vi "DestroyRenderer.vi"(8 "No Error":errorcluster, 11 "Rrenderer [SDL_Renderer *]":i64 format="%.0x") -> (0 "error out":errorcluster)   [LabVIEW 2024, in "SDL3.lvlib" / "Render.lvlib"]
doc: "<B>Summary</B>\nDestroy the rendering context for a window and free all associated textures.\n\n<B>Remarks</B>\nThis should be called before destroying the associated window."
uses:
  Render.lvlib
  Lib/Win32/SDL3.dll
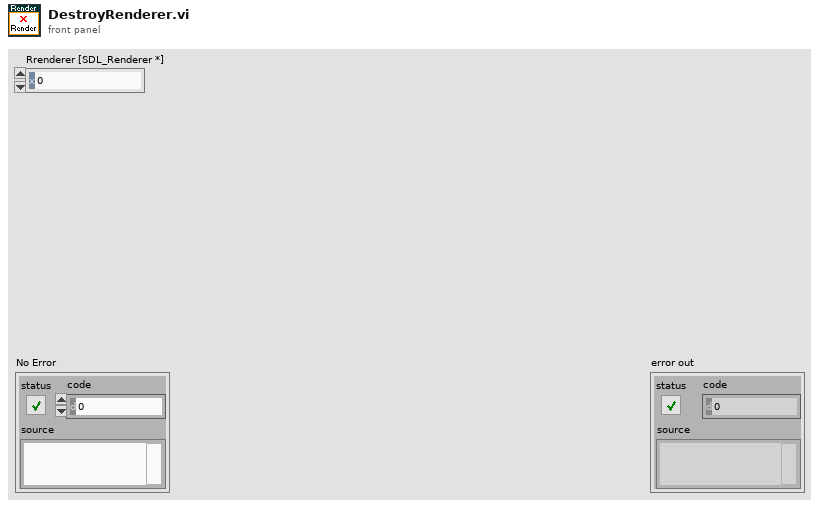
[diagram p1: front panel]
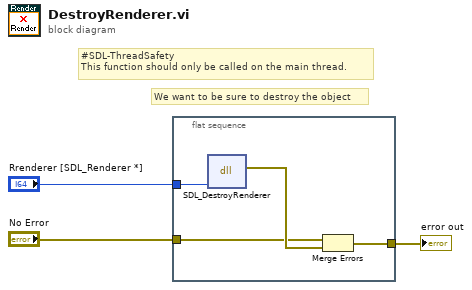
[diagram p0: block diagram]
diagram:
  # "#SDL-ThreadSafety\nThis function should only be called on the main thread."
  # "We want to be sure to destroy the object"
  n1 = flat-sequence {
    tunnel: [w6] -> w3
    tunnel: "No Error" -> [w5]
    tunnel: "Rrenderer [SDL_Renderer *]" -> [w4]
    frame #0 {
      n2 = dll-call lib="C:/Users/Thomas/Documents/Projects/LV-SDL3/Lib/Win32/SDL3.dll" fn="SDL_DestroyRenderer"("window"=w4) -> (error out=w7:errorcluster)  [unwired: 5 in, 1 out]
      n3 = Merge Errors(w5, w7) -> (w6:errorcluster)
    }
  }
  "error out" <- w3
